vi "lo export.vi"(8 "error in (no error)":errorcluster, 9 "filename":string, 10 "lobjId":u32) -> (0 "error out":errorcluster, 2 "lo_export":i32)   [LabVIEW 2019, in "libpqlv.lvlib"]
uses:
  libpqlv.lvlib
  libpq.dll
panel:
  in  "conn":u32
  out "conn_out":u32
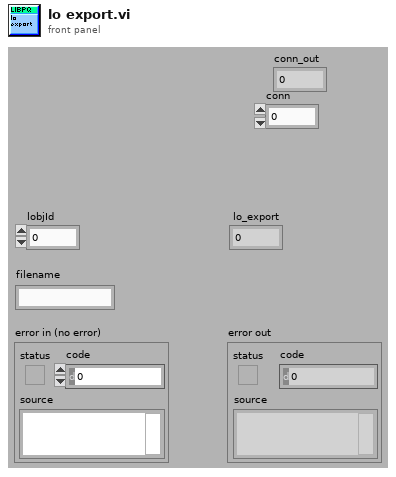
[diagram p1: front panel]
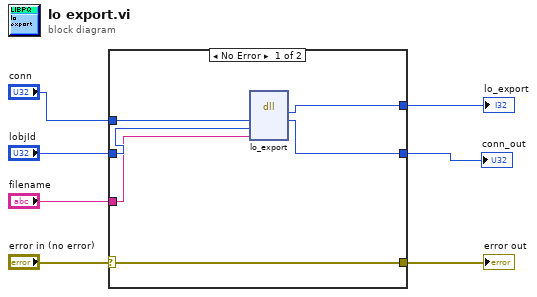
[diagram p0: block diagram]
diagram:
  n1 = case shown="No Error" "error in (no error)" {
    selector: "error in (no error)" -> [w13 w15]
    tunnel: [w13 w15] -> w6
    tunnel: [w12 _] -> w5
    tunnel: [w11 w14] -> w2
    tunnel: "lobjId" -> [w10 _]
    tunnel: "filename" -> [w9 _]
    tunnel: "conn" -> [w8 w14]
    frame No Error {
      n2 = dll-call lib="libpq.*" fn="lo_export"("conn"=w8, "lobjId"=w10, "filename"=w9) -> ("lo_export"=w12:i32, "conn"=w11:u32)  [unwired: 5 in, 2 out]
    }
    frame Error {
    }
  }
  "lo_export" <- w5
  "error out" <- w6
  "conn_out" <- w2
